vi "ster kartezjan.vi"(0 "Digital in":refnum<vi>, 1 "Numeric 5":dbl, 2 "reference 2":refnum<vi>, 3 "reference":refnum<vi>, 4 "Numeric 2":dbl, 6 "Sterowanie w ukladzie narzêdzia":bool, 7 "Numeric":dbl) -> (8 "q1":dbl format="%.2f", 9 "Py":dbl(slide) scale=0.0..1075.0, 10 "q2":dbl format="%.2f", 11 "Pz":dbl(slide) scale=0.0..1149.0, 12 "q3":dbl format="%.2f", 13 "Px":dbl(slide) scale=0.0..1075.0, 14 "Numeric 6":dbl, 15 "Numeric 4":dbl, 16 "q4":dbl format="%.2f", 17 "Numeric 3":dbl, 18 "q5":dbl format="%.2f")   [LabVIEW 2014]
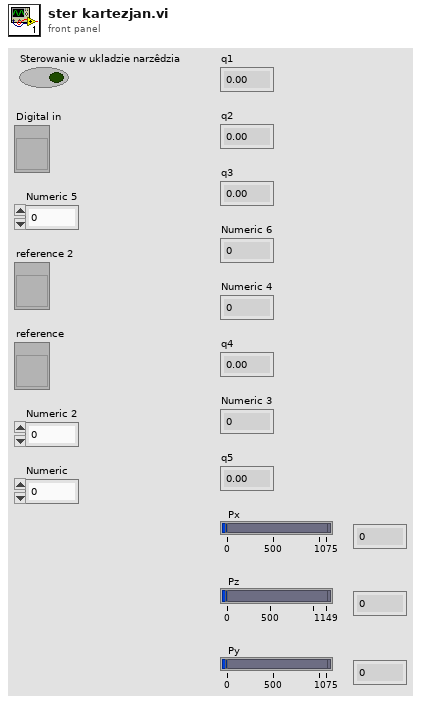
[diagram p1: front panel]
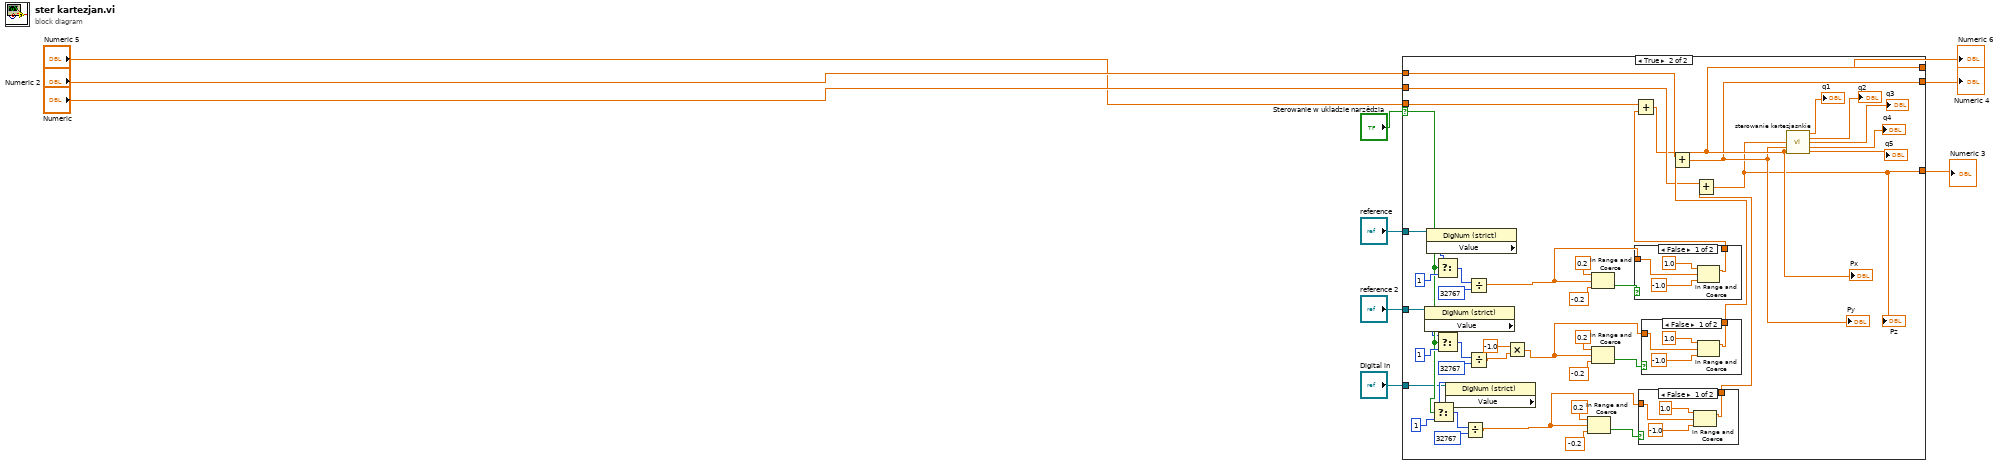
[diagram p0: block diagram]
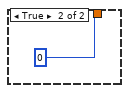
[diagram p3: hidden frame]
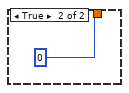
[diagram p4: hidden frame]
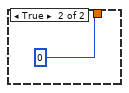
[diagram p5: hidden frame]
diagram:
  n1 = case shown="True" "Sterowanie w ukladzie narzêdzia" {
    selector: "Sterowanie w ukladzie narzêdzia" -> [_ w29]
    tunnel: [w13 w26] -> w4
    tunnel: "Numeric 5" -> [w13 w44]
    tunnel: [w12 w25] -> w7
    tunnel: [w11 w24] -> w8
    tunnel: "Numeric 2" -> [w12 w28]
    tunnel: "Numeric" -> [w11 w27]
    tunnel: "reference" -> [_ w16]
    tunnel: "reference 2" -> [_ w15]
    tunnel: "Digital in" -> [_ w14]
    frame False {
    }
    frame True {
      n2 = property class="DigNum (strict)"(reference=w15) -> ("Value"=w23:i32)  [unwired: 1 in, 2 out]
      n3 = property class="DigNum (strict)"(reference=w16) -> ("Value"=w46:i32)  [unwired: 1 in, 2 out]
      n4 = Select(t=w46, s=w29, f=1) -> (s? t:f=w48:i32)
      n5 = Select(t=w23, s=w29, f=1) -> (s? t:f=w42:i32)
      n6 = property class="DigNum (strict)"(reference=w14) -> ("Value"=w22:i32)  [unwired: 1 in, 2 out]
      n7 = Select(t=w22, s=w29, f=1) -> (s? t:f=w33:i32)
      n8 = Divide(x=w33, y=32767) -> (x/y=w20:dbl)
      n9 = Divide(x=w48, y=32767) -> (x/y=w21:dbl)
      n10 = Divide(x=w42, y=32767) -> (x/y=w18:dbl)
      n11 = Multiply(x=-1.0, y=w18) -> (x*y=w17:dbl)
      n12 = In Range and Coerce(upper limit=0.2 ("y"), x=w20, lower limit=-0.2 ("y")) -> (In Range?=w32:bool)  [unwired: 1 out]
      n13 = In Range and Coerce(upper limit=0.2 ("y"), x=w21, lower limit=-0.2 ("y")) -> (In Range?=w47:bool)  [unwired: 1 out]
      n14 = In Range and Coerce(upper limit=0.2 ("y"), x=w17, lower limit=-0.2 ("y")) -> (In Range?=w43:bool)  [unwired: 1 out]
      n15 = case shown="False" w47 {
        tunnel: [w69 0 ("y")] -> w45
        tunnel: w21 -> [w68 _]
        frame False {
          n16 = In Range and Coerce(upper limit=1.0 ("y"), x=w68, lower limit=-1.0 ("y")) -> (coerced(x)=w69:dbl)  [unwired: 1 out]
        }
        frame True {
        }
      }
      n17 = Add(x=w44, y=w45) -> (x+y=w26:dbl)
      "Px" <- w26
      n18 = case shown="False" w32 {
        tunnel: [w59 0 ("y")] -> w30
        tunnel: w20 -> [w58 _]
        frame False {
          n19 = In Range and Coerce(upper limit=1.0 ("y"), x=w58, lower limit=-1.0 ("y")) -> (coerced(x)=w59:dbl)  [unwired: 1 out]
        }
        frame True {
        }
      }
      n20 = case shown="False" w43 {
        tunnel: [w64 0 ("y")] -> w31
        tunnel: w17 -> [w63 _]
        frame False {
          n21 = In Range and Coerce(upper limit=1.0 ("y"), x=w63, lower limit=-1.0 ("y")) -> (coerced(x)=w64:dbl)  [unwired: 1 out]
        }
        frame True {
        }
      }
      n22 = Add(x=w28, y=w31) -> (x+y=w25:dbl)
      "Py" <- w25
      n23 = Add(x=w27, y=w30) -> (x+y=w24:dbl)
      "Pz" <- w24
      n24 = call "sterowanie kartezjasnkie.vi"("Pz"=w24, "Py"=w25, "Px"=w26) -> ("q1"=→"q1":dbl, "q2"=→"q2":dbl, "q3"=→"q3":dbl, "q4"=→"q4":dbl, "q5"=→"q5":dbl)  [unwired: 8 in]
    }
  }
  "Numeric 3" <- w8
  "Numeric 4" <- w7
  "Numeric 6" <- w4
